vi "Update.vi"(8 "error in (no error)":errorcluster, 11 "Tetris in":refnum<class "Tetris.lvclass">) -> (0 "error out":errorcluster, 3 "Tetris out":refnum<class "Tetris.lvclass">)   [LabVIEW 2019, in "RT_Game.lvlib" / "Tetris.lvclass"]
uses:
  Tetris.lvclass
  Game/Game.lvclass
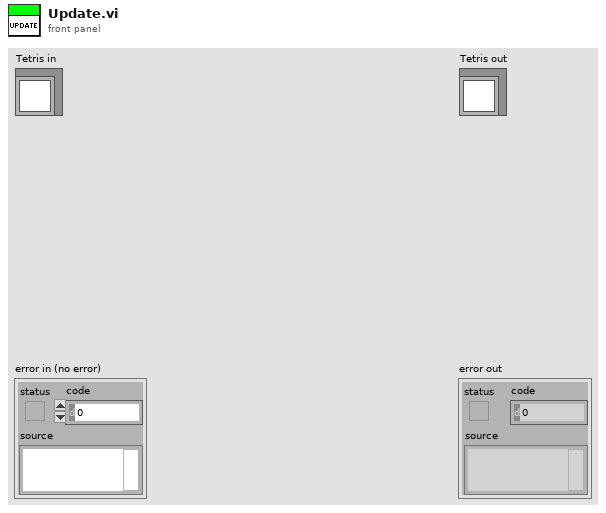
[diagram p1: front panel]
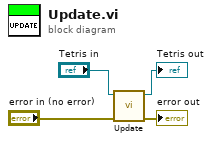
[diagram p0: block diagram]
diagram:
  n1 = call-parent "Update.vi"("error in (no error)"="error in (no error)", "Game in"="Tetris in") -> ("error out"=→"error out":errorcluster, "Game out"=→"Tetris out":refnum<class "Tetris.lvclass">)  [unwired: 8 in]
